vi "KepcoDCPwr Configure User Sequence.vi"(0 "VISA Session":refnum<visa-resource-name>, 1 "List Mode (volt/current)":enum16{"Current List", "Voltage List"}(ring), 5 "Model In":string, 7 "channel name (\"\")":string="\"\"", 9 "# of Cycles":i32=1 min=0 max=255, 11 "error in (no error)":errorcluster {"code" format="%.0x"}, 12 "Dwell (sec)":dbl[](array[numeric]) format="%.4f", 13 "List Data":dbl[](array[numeric]) format="%.2f", 14 "Limit Value":dbl format="%.2f") -> (4 "VISA Session Out":refnum<visa-resource-name>, 6 "Model Out":string, 8 "channel name out (\"\")":string="\"\"" caption="channel name Out (\"\")", 15 "error out":errorcluster {"code" format="%.0x"})   [LabVIEW 2020]
doc: "This VI configures the user list sequence.\nIt clears any existing list, initalizes the alternate channel correctly based upon model\ndownloads the list array\ndownads the dwell array or single entry for all dewlls.\n\nThis VI is designed following best pratice operation, i.e only main channel is initalized \n\nIts inputs are multiple points of eather voltage or current. Single dwell point, single limit point.\n\nProvides count and list mode inputs."
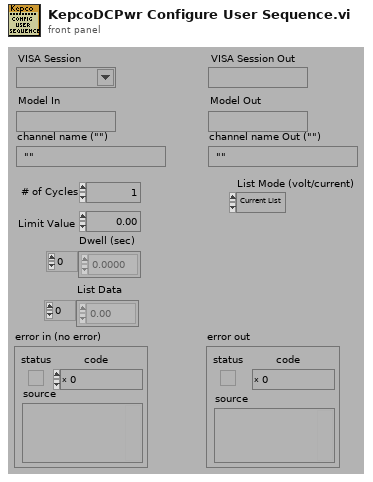
[diagram p1: front panel]
types:
  T1 = enum16{"Current List", "Voltage List", "DWell List"}
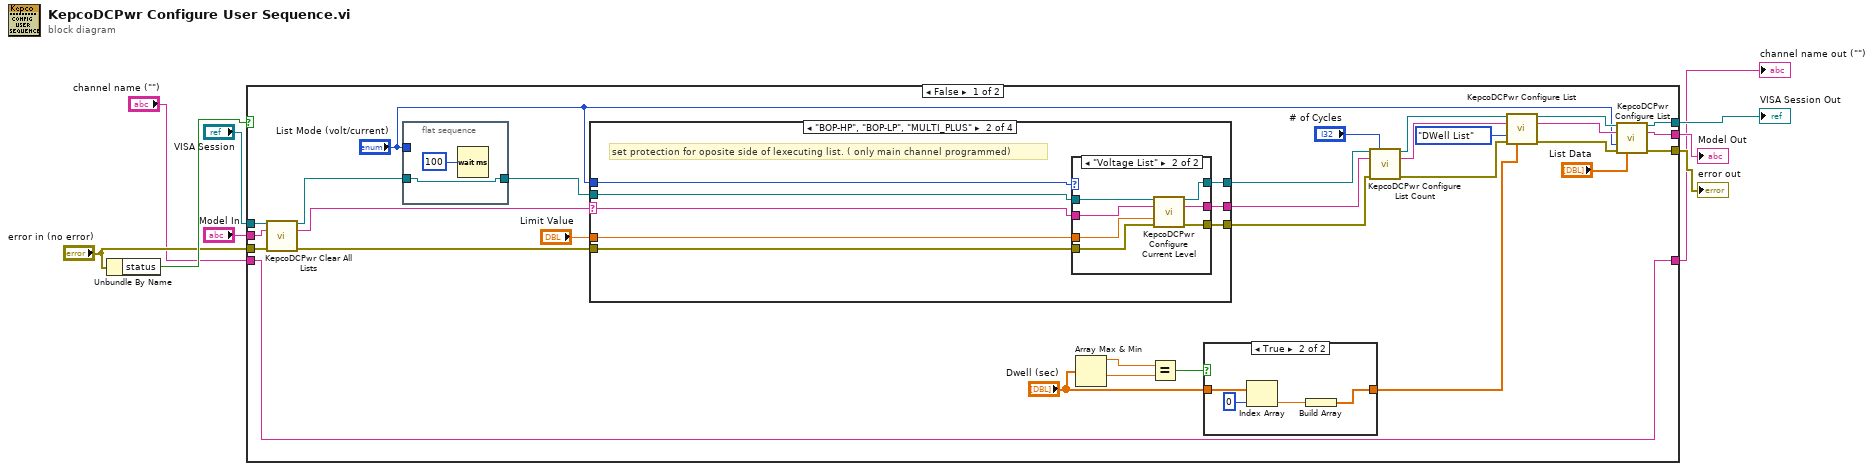
[diagram p0: block diagram]
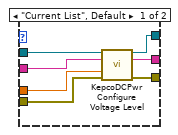
[diagram p4: hidden frame]
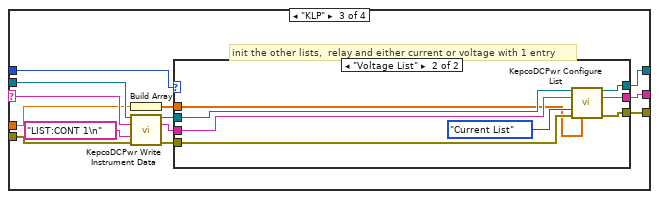
[diagram p5: hidden frame]
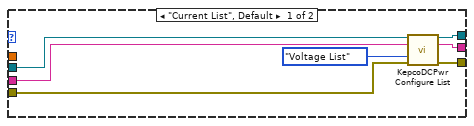
[diagram p6: hidden frame]
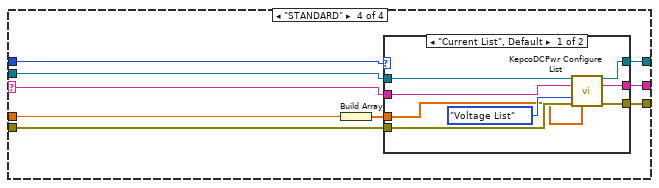
[diagram p7: hidden frame]
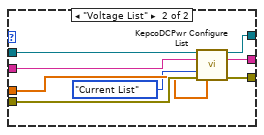
[diagram p8: hidden frame]
diagram:
  n1 = Unbundle By Name("error in (no error)") -> ("status"=w8:bool)
  n2 = case shown="False" w8 {
    tunnel: [w33 w128] -> w9
    tunnel: "error in (no error)" -> [w10 w128]
    tunnel: "VISA Session" -> [w12 w127]
    tunnel: "Model In" -> [w11 w126]
    tunnel: "channel name (\"\")" -> [w39 w125]
    tunnel: [w31 w127] -> w3
    tunnel: [w32 w126] -> w2
    tunnel: [w39 w125] -> w1
    frame False {
      n3 = call "KepcoDCPwr Clear All Lists.vi"("VISA Session"=w12, "Model In"=w11, "error in (no error)"=w10) -> ("VISA Session Out"=w13:refnum<visa-resource-name>, "Model Out"=w14:string, "error out"=w15:errorcluster)  [unwired: 9 in, 1 out]
      n4 = flat-sequence {
        tunnel: w13 -> [w41]
        tunnel: [w41] -> w24
        tunnel: "List Mode (volt/current)" -> [_]
        frame #0 {
          n5 = Wait (ms)(milliseconds to wait=u32 100) -> ()  [unwired: 1 out]
        }
      }
      n6 = case shown="\"BOP-HP\", \"BOP-LP\", \"MULTI_PLUS\"" w14 {
        selector: w14 -> [w48 w55 w82 w105]
        tunnel: [w49 w56 w79 w107] -> w20
        tunnel: w15 -> [w49 w57 w83 w108]
        tunnel: [w48 w54 w77 w106] -> w19
        tunnel: w24 -> [w47 w53 w81 w103]
        tunnel: [w47 w52 w75 w104] -> w18
        tunnel: "Limit Value" -> [_ w51 w73 w101]
        tunnel: "List Mode (volt/current)" -> [_ w50 w72 w100]
        frame "", "MULTI", Default {
        }
        frame "BOP-HP", "BOP-LP", "MULTI_PLUS" {
          # "set protection for oposite side of lexecuting list. ( only main channel programmed)"
          n7 = case shown="\"Voltage List\"" w50 {
            tunnel: w57 -> [w61 w71]
            tunnel: [w62 w70] -> w56
            tunnel: w55 -> [w58 w69]
            tunnel: [w64 w68] -> w54
            tunnel: w53 -> [w60 w67]
            tunnel: [w63 w66] -> w52
            tunnel: w51 -> [w59 w65]
            frame "Current List", Default {
              n8 = call "KepcoDCPwr Configure Voltage Level.vi"("VISA Session"=w60, "Model In"=w58, "level (0.0 volts)"=w59, "error in (no error)"=w61) -> ("VISA Session Out"=w63:refnum<visa-resource-name>, "Model Out"=w64:string, "error out"=w62:errorcluster)  [unwired: 8 in, 1 out]
            }
            frame "Voltage List" {
              n9 = call "KepcoDCPwr Configure Current Level.vi"("VISA Session"=w67, "Model In"=w69, "level (0.0 volts)"=w65, "error in (no error)"=w71) -> ("VISA Session Out"=w66:refnum<visa-resource-name>, "Model Out"=w68:string, "error out"=w70:errorcluster)  [unwired: 1 in, 8 out]
            }
          }
        }
        frame "KLP" {
          # "init the other lists,  relay and either current or voltage with 1 entry"
          n10 = Build Array(w73) -> (w74:dbl[])
          n11 = call "KepcoDCPwr Write Instrument Data.vi"("VISA Session"=w81, "Model"=w82, "Write Buffer"="LIST:CONT 1\n", "error in (no error)"=w83) -> ("VISA Session Out"=w76:refnum<visa-resource-name>, "Model Out"=w78:string, "error out"=w80:errorcluster)  [unwired: 1 in, 8 out]
          n12 = case shown="\"Voltage List\"" w72 {
            tunnel: w80 -> [w90 w99]
            tunnel: [w87 w98] -> w79
            tunnel: w78 -> [w89 w97]
            tunnel: [w86 w96] -> w77
            tunnel: w76 -> [w85 w95]
            tunnel: [w88 w94] -> w75
            tunnel: w74 -> [_ w92]
            frame "Current List", Default {
              n13 = call "KepcoDCPwr Configure List.vi"("VISA Session"=w85, "Model In"=w89, "List Type (DWell)"=T1."Voltage List", "error in (no error)"=w90) -> ("VISA Session Out"=w88:refnum<visa-resource-name>, "Model Out"=w86:string, "error out"=w87:errorcluster)  [unwired: 2 in, 7 out]
            }
            frame "Voltage List" {
              n14 = call "KepcoDCPwr Configure List.vi"("VISA Session"=w95, "Model In"=w97, "List Type (DWell)"=T1."Current List", "error in (no error)"=w99, "List"=w92) -> ("VISA Session Out"=w94:refnum<visa-resource-name>, "Model Out"=w96:string, "error out"=w98:errorcluster)  [unwired: 1 in, 7 out]
            }
          }
        }
        frame "STANDARD" {
          n15 = Build Array(w101) -> (w102:dbl[])
          n16 = case shown="\"Current List\", Default" w100 {
            tunnel: w108 -> [w112 w124]
            tunnel: [w113 w123] -> w107
            tunnel: [w114 w122] -> w106
            tunnel: w105 -> [w111 w121]
            tunnel: [w115 w120] -> w104
            tunnel: w103 -> [w110 w119]
            tunnel: w102 -> [w109 w118]
            frame "Current List", Default {
              n17 = call "KepcoDCPwr Configure List.vi"("VISA Session"=w110, "Model In"=w111, "List Type (DWell)"=T1."Voltage List", "error in (no error)"=w112, "List"=w109) -> ("VISA Session Out"=w115:refnum<visa-resource-name>, "Model Out"=w114:string, "error out"=w113:errorcluster)  [unwired: 1 in, 7 out]
            }
            frame "Voltage List" {
              n18 = call "KepcoDCPwr Configure List.vi"("VISA Session"=w119, "Model In"=w121, "List Type (DWell)"=T1."Current List", "error in (no error)"=w124, "List"=w118) -> ("VISA Session Out"=w120:refnum<visa-resource-name>, "Model Out"=w122:string, "error out"=w123:errorcluster)  [unwired: 1 in, 7 out]
            }
          }
        }
      }
      n19 = Array Max & Min(array="Dwell (sec)") -> (max value=w29:dbl, min value=w28:dbl)  [unwired: 2 out]
      n20 = Equal?(x=w29, y=w28) -> (x = y?=w27:bool)
      n21 = case shown="True" w27 {
        tunnel: "Dwell (sec)" -> [w42 w46]
        tunnel: [w42 w43] -> w25
        frame False {
        }
        frame True {
          n22 = Index Array(array=w46, index=0) -> (element=w44:dbl)
          n23 = Build Array(w44) -> (w43:dbl[])
        }
      }
      n24 = call "KepcoDCPwr Configure List Count.vi"("VISA Session"=w18, "# of Cycles"="# of Cycles", "Model In"=w19, "error in (no error)"=w20) -> ("VISA Session Out"=w21:refnum<visa-resource-name>, "Model Out"=w17:string, "error out"=w16:errorcluster)  [unwired: 8 in, 1 out]
      n25 = call "KepcoDCPwr Configure List.vi"("VISA Session"=w21, "Model In"=w17, "List Type (DWell)"=T1."DWell List", "error in (no error)"=w16, "List"=w25) -> ("VISA Session Out"=w37:refnum<visa-resource-name>, "Model Out"=w36:string, "error out"=w35:errorcluster)  [unwired: 1 in, 7 out]
      n26 = call "KepcoDCPwr Configure List.vi"("VISA Session"=w37, "Model In"=w36, "List Type (DWell)"="List Mode (volt/current)", "error in (no error)"=w35, "List"="List Data") -> ("VISA Session Out"=w31:refnum<visa-resource-name>, "Model Out"=w32:string, "error out"=w33:errorcluster)  [unwired: 1 in, 7 out]
    }
    frame True {
    }
  }
  "error out" <- w9
  "channel name out (\"\")" <- w1
  "Model Out" <- w2
  "VISA Session Out" <- w3
